vi "TransferCavityLock_InfIntegral_SlowCavityLock.vi"() -> ()   [LabVIEW 2016]
uses:
  <vilib>/DAQmx/read.llb/DAQmx Read (Analog 1D Wfm NChan NSamp Duration).vi
  <vilib>/Analysis/baseanly.llb/Mean (DBL).vi
  <vilib>/DAQmx/create/channels.llb/DAQmx Create Channel (AI-Voltage-Basic).vi
  <vilib>/DAQmx/configure/timing.llb/DAQmx Timing (Sample Clock).vi
  <vilib>/DAQmx/configure/trigger.llb/DAQmx Start Trigger (Digital Edge).vi
  <vilib>/DAQmx/miscellaneous.llb/DAQmx Fill In Error Info.vi
  <vilib>/Waveform/WDTOps.llb/WDT Get Waveform Subset DBL.vi
  <vilib>/measure/mamon.llb/Waveform Peak Detection for 1 Chan.vi
  <vilib>/addons/control/pid/pid.llb/PID (DBL).vi
  <vilib>/measure/NI_MAPro.lvlib
  <vilib>/Analysis/NI_AALBase.lvlib
  <vilib>/addons/control/pid/NI_PID_pid.lvlib
  <vilib>/gmath/NI_Gmath.lvlib
panel:
  in  "Limit for cavity lock":bool
  in  "Polarity 2":i8=1 min=-1 max=1 step=2
  in  "Polarity 1":i8=1 min=-1 max=1 step=2
  out "Integral for cavity lock":dbl=0.008257081575736186 format="%0.5f V"
  out "Cavity scan offset Output":dbl=3.2082570815757308 min=0.0 step=0.01 format="%.5f V"
  in  "Cavity scan offset":dbl=3.1999999999999944 min=0.0 step=0.01 format="%.5f V"
  in  "OK Button 2":bool
  out "Error Signal for cavity lock":dbl(graph)=1.2838768115943822
  in  "Setpoint for cavity lock":dbl=1950.0 min=0.0 step=0.1 format="%.2f"
  in  "I Factor for cavity lock":dbl=5e-05 min=0.0 step=1e-05 format="%.5f"
  out "Peak Loc2":dbl(graph)=2256.4418259303447
  out "Peak Loc1":dbl(graph)=1948.7161231884056
  out "PZT Output":dbl(graph)=4.680700597703368
  out "Noise Std":dbl=0.03727411119636263 format="%0.3f V"
  out "size(s)":i32=100
  out "Histogram":dynamicdata(graph)=[{"t0"=timestamp(-0.09499999999999997 s since 1904-01-01), "dt"=0.01, "Y"=[0.6724792202903564, 0.8210147212924623, 2.0418544555563467, 2.399967444273753, 2.6421006582360897, 3.8191936353555187, 6.9191091939405664, 9.895923412654003, 9.585626646861932, 10.44733602596319, 14.545288067308965, 9.500167865463462, 6.621020825491134, 7.961909800290967, 3.825297834026838, 3.17316594264088, 2.0886533120364623, 1.9238399479108381, 0.4415370372254382, 0.6745139531807962], "attributes"=variant("NI_ChannelName"=variant(string " (Histogram)"), "NI_ExpIsRelativeTime"=variant(bool TRUE), "NI_ExpStartTimeStamp"=variant(timestamp timestamp(0 s since 1904-01-01)), "NI_ExpTimeStamp"=variant(timestamp timestamp(0 s since 1904-01-01)), "NI_ExpXDimension"=variant(string "BIN"), "NI_OriginalChannelName"=variant(string ""))}]
  out "Integral":dbl=-0.31929940229663345 format="%0.3f V"
  in  "I Factor":dbl=0.06 min=0.0 step=1e-05 format="%.3f"
  in  "Proportional":T1={"Proportional gain (Kc)"=0.005, "Integral time (Ti, min)"=0.1, "Derivative time (Td, min)"=0.0} {"Derivative time (Td, min)" min=0.0 step=0.1 format="%.2f"; "Integral time (Ti, min)" min=0.0 step=0.1 format="%.2f"; "Proportional gain (Kc)" min=0.0 step=0.1 format="%.3f"}
  out "P Array":dbl[](array[numeric])=[0.06979206777050706, -0.06757152621814555, 0.0253521126760603, 0.04560439560439988, -0.038277511961723576, 0.036986301369879016, -0.04494569757727618, 0.02419763085957527, 0.018115942028984477, -0.011801242236018084, -0.012648809523824411, -0.04897959183674061, 0.023401360544227146, -0.007827788649706235, -0.02202273314389913, 0.011767925561031234, 0.011688311688303088, -0.023990241257791922, -0.02863234846175544, 0.06390977443608392, -0.052721088435390584, 0.057637600494757635, 0.03265306122450795, 0.08333333333334281, -0.014731645166421004, -9.5174645480256e-05, 0.00201465201466533, -0.1062769282757472, 0.06927854753941176, -0.010158730158735807, 0.03962304562004704, -0.08253968253968935, -0.058129809300780266, -0.06380952380952465, 0.056462585033997925, 0.010964912280698513, 0.006632653061231508, 0.09833024118738365, -0.03107769423559148, 0.02233831742027803, -0.031212484993986322, 0.005787389582692981, 0.03754094230284011, 0.08456760630672022, 0.01198879551820653, -0.020408163265315693, 0.002782931354346374, 0.005864661654143788, -0.029870129870133155, 0.009480715363082481, -0.07006573673240268, -0.01208244491826349, -0.018367346938788387, -0.04200542005420971, -0.041410488245915644, 0.0015444015443932813, 0.009890109890108079, -0.05175983436853926, -0.017460317460304964, -0.015971606033730268, 0.0018796992481213692, -0.03761904761904589, -0.03679653679652972, 0.040224785566394416, 0.022408963585434094, 0.009680795395070163, 0.11904761904760619, 0.01256157635468469, 0.00023060071485758726, -0.027777777777785673, -0.03336594911937141, 0.034962406015054626, -0.040259740259742216, -0.030677655677649796, 0.01959183673470477, -0.02309092651145761, -0.0007963051441350899, -0.0, -0.0, -0.0, 0.0, -0.0, -0.0, 0.0, 0.0, 0.0, -0.0, 0.0, -0.0, 0.0, 0.0, 0.0, 0.0, -0.0, 0.0, -0.0, -0.0, -0.0, 0.0, -0.0]
  out "Full?":bool=TRUE
  in  "PZT Value":dbl=5.000000000000002 min=0.0 step=0.01 format="%.2f V"
  out "Error Signal":dbl(graph)=-0.003649068322971516
  in  "Output Range":cluster{"Output high":dbl, "Output low":dbl}={"Output high"=1.0, "Output low"=-1.0} {"Output low" min=0.0 format="%.2f"; "Output high" min=0.0 max=1.0 format="%.2f"}
  out "P Output":dbl=-1.824534161485758e-05 format="%0.3f V"
  in  "Setpoint":dbl=115.0 min=0.0 step=0.1 format="%.2f"
  out "dt out (s)":dbl=0.4020000190939754 format="%.3f"
  out "Number of Peaks":i32=8
  out "Average Spacing":dbl(graph)=115.00364906832297
  out "Current Value":dbl=115.00364906832297 format="%0.2f"
  out "Spcaing":dbl[](array[numeric])=[58.58871915393655, 185.2243243243243, 71.53859649122808, 165.22807017543857, 82.54838709677426, 146.8474462365591, 95.04999999999995]
  out "Locations":dbl[](array[numeric])=[128.58695652173913, 187.17567567567568, 372.4, 443.93859649122805, 609.1666666666666, 691.7150537634409, 838.5625, 933.6125]
  out "error out 2":errorcluster
  in  "Peak Thres":dbl=-0.15 format="%.2f"
  in  "width 2":i32=3 min=3
  out "Waveform Graph 2":waveform(dbl)(graph)={"t0"=timestamp(3654386435.809387 s since 1904-01-01), "dt"=9.999999999999999e-05, "Y"=array[1000 elements], "attributes"=variant("NI_ChannelName"=variant(string "Voltage_1"), "NI_UnitDescription"=variant(string "Volts"))}
  out "Rate":dbl=5.0 format="%#_g Hz"
  in  "OK Button":bool
  in  "Physical channels":tag="Dev1/ao0"
  out "Waveform Graph":waveform(dbl)[](graph)=[{"t0"=timestamp(3654386435.7613373 s since 1904-01-01), "dt"=9.999999999999999e-05, "Y"=array[1500 elements], "attributes"=variant("NI_ChannelName"=variant(string "Voltage_0"), "NI_UnitDescription"=variant(string "Volts"))}, {"t0"=timestamp(3654386435.7613873 s since 1904-01-01), "dt"=9.999999999999999e-05, "Y"=array[1500 elements], "attributes"=variant("NI_ChannelName"=variant(string "Voltage_1"), "NI_UnitDescription"=variant(string "Volts"))}]
  in  "error in":errorcluster
  in  "stop":bool
  # "锁定：\n1. Proportional gain (Kc)设置为0.005\n2. Integral time (Ti, min)设置为0.10\n3. Derivative time (Td, min)设置为0.00\n4. I Factor设置为0.06\n5. 调节PZT电压使得Current Value在Setpoint附近（Error Signal0.1以内）\n6. 点击Lock Off，状态变为Lock On \n\n解锁：\n1. 点击Lock On\n2. 点击Stop"
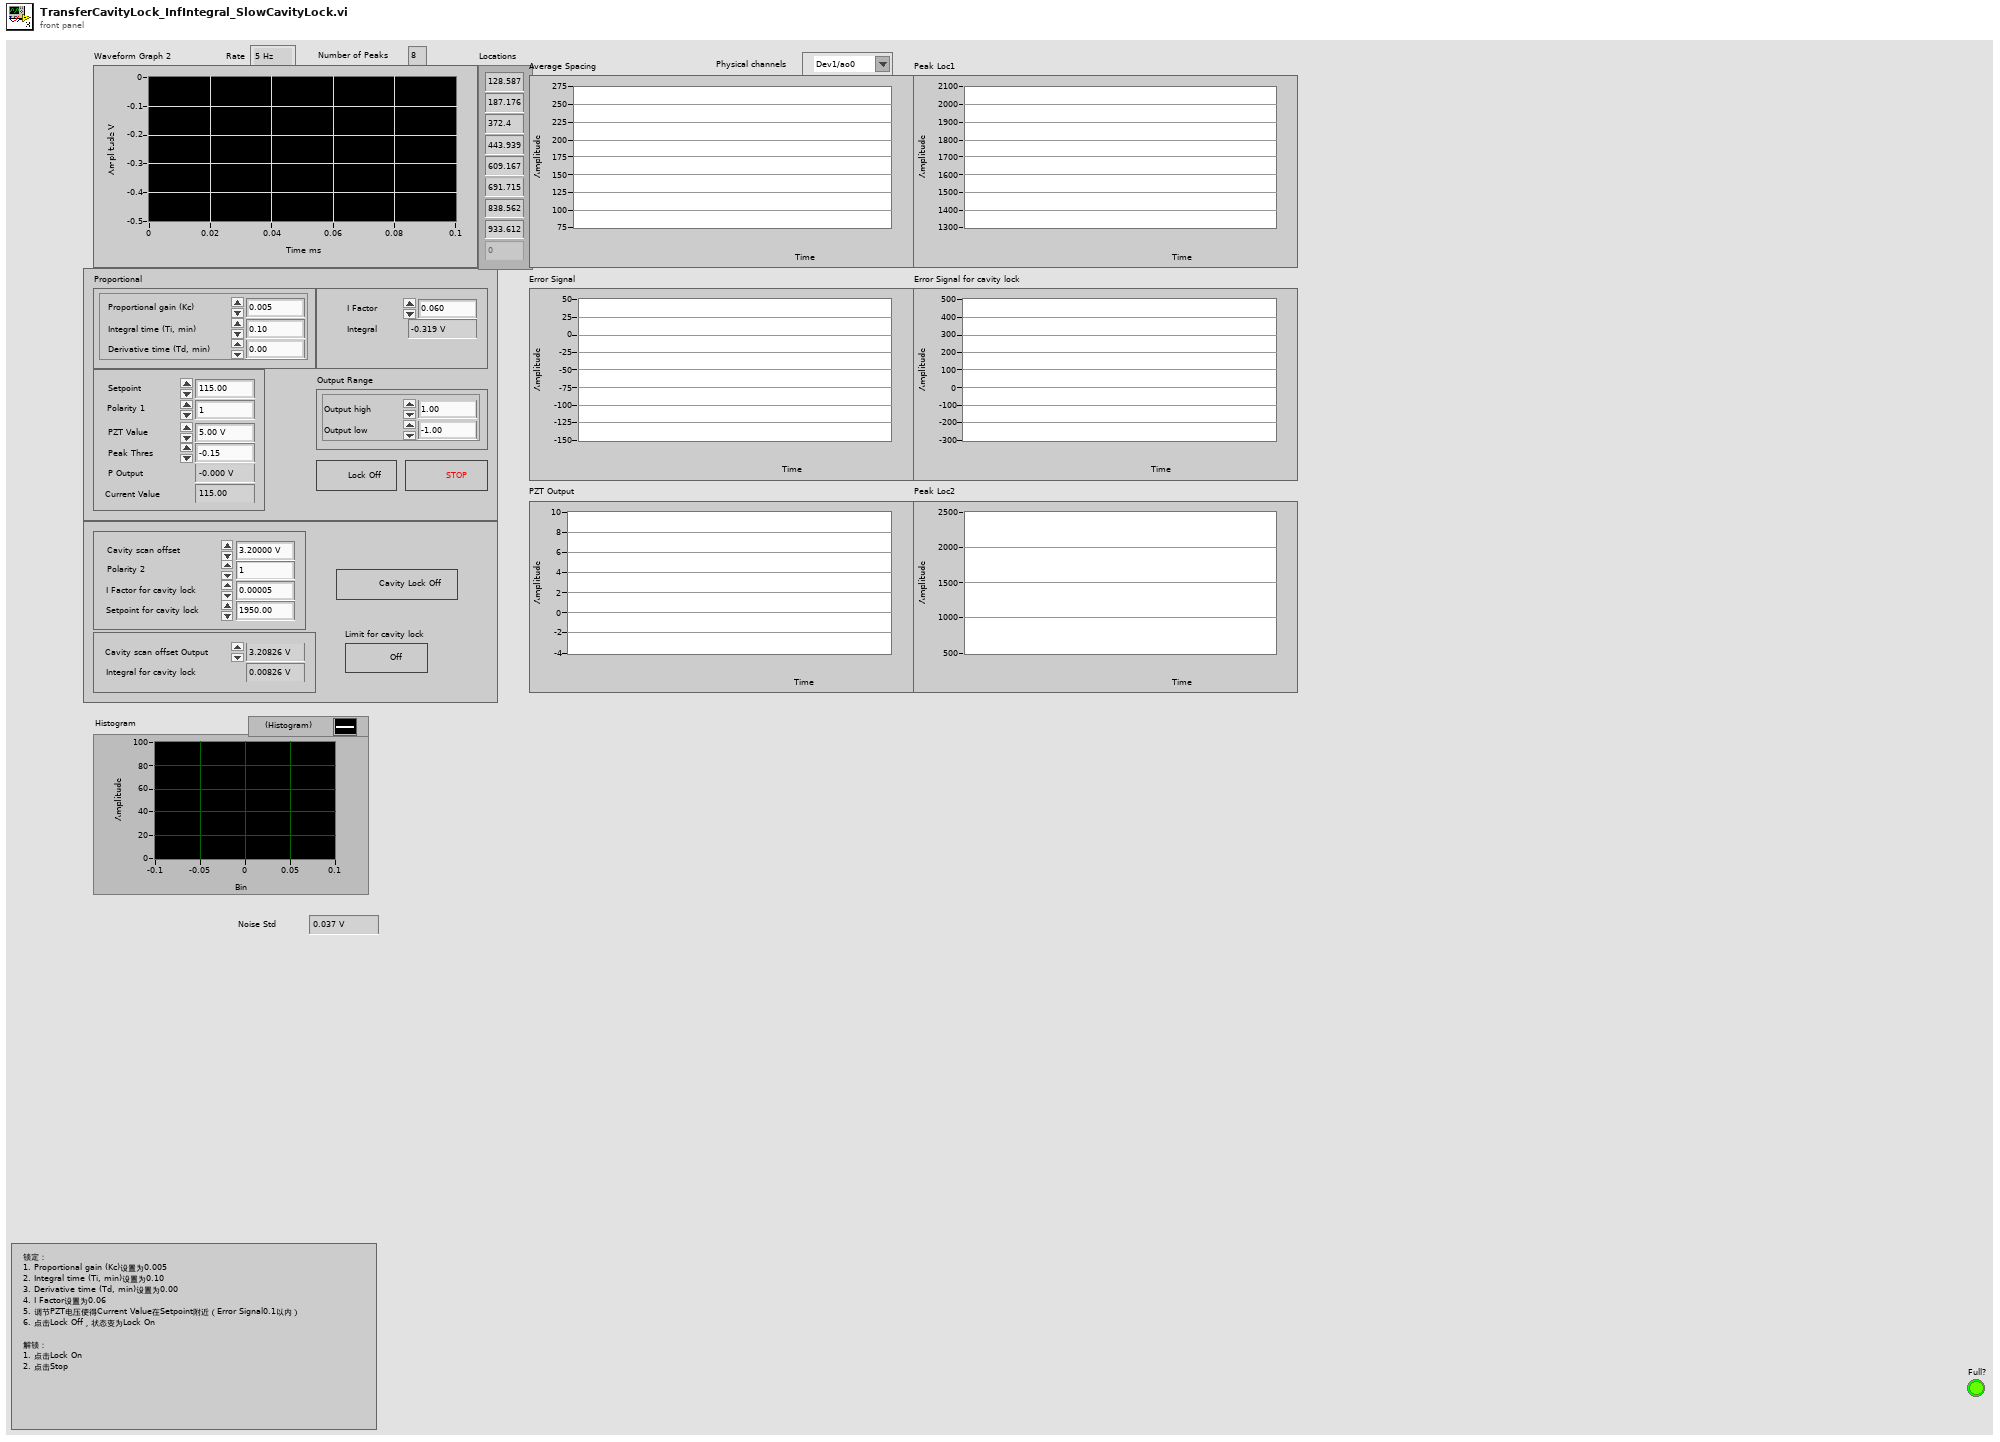
[diagram p1: front panel]
types:
  T1 = cluster{"Proportional gain (Kc)":dbl, "Integral time (Ti, min)":dbl, "Derivative time (Td, min)":dbl}
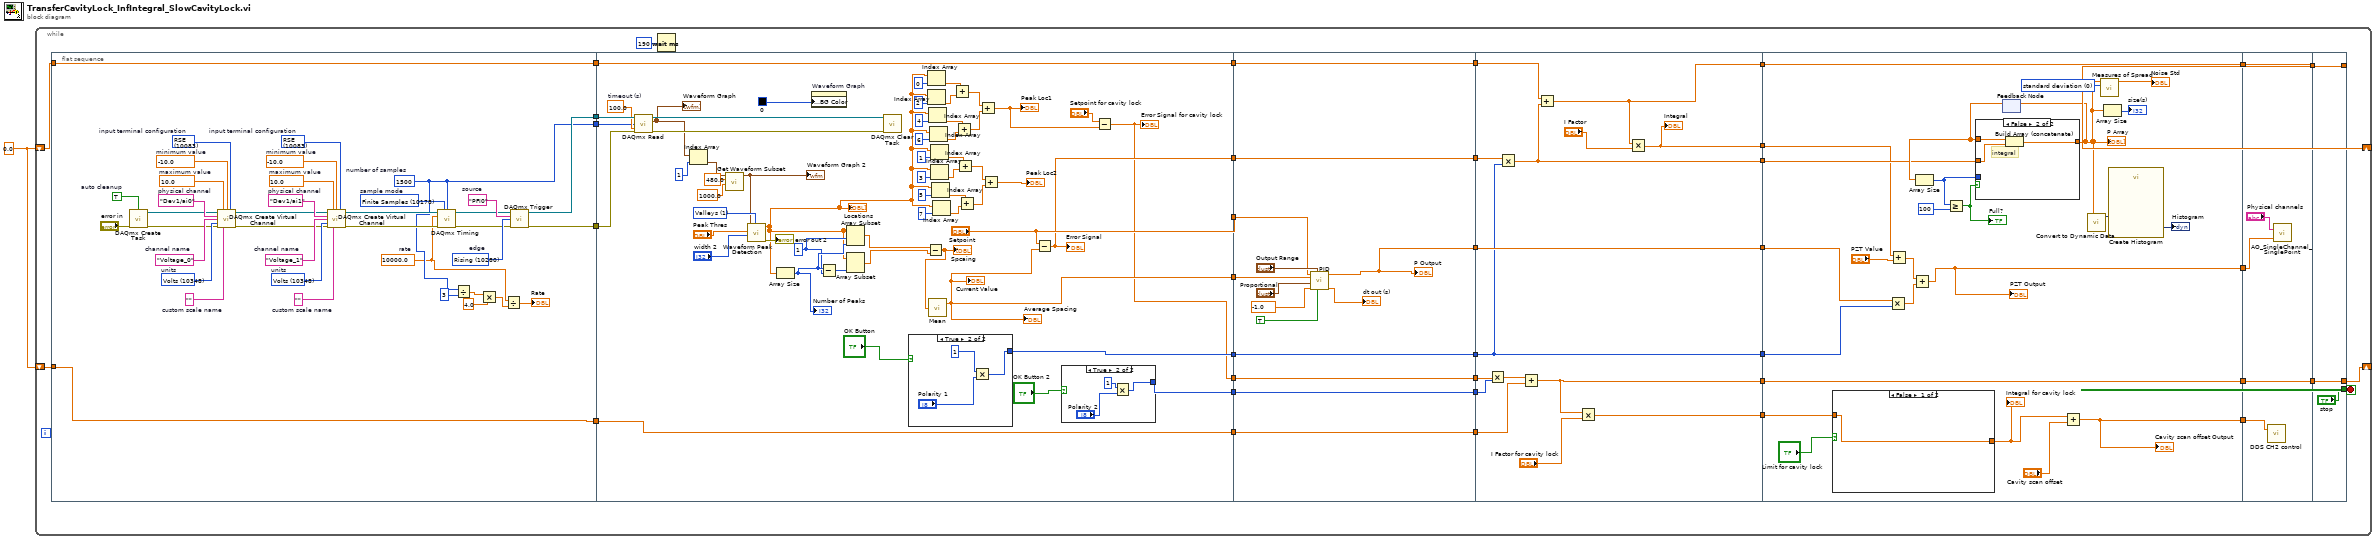
[diagram p0: block diagram]
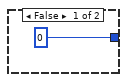
[diagram p2: hidden frame]
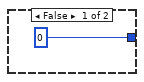
[diagram p3: hidden frame]
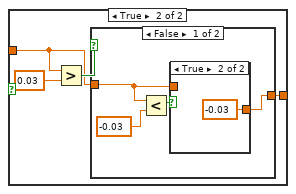
[diagram p4: hidden frame]
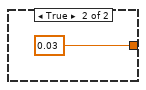
[diagram p6: hidden frame]
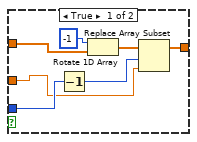
[diagram p7: hidden frame]
diagram:
  w1 = 0.0
  n1 = while {
    shift-right: [w17] -> _
    shift-left: w1 -> [w23]
    shift-right: [w2] -> _
    shift-left: w1 -> [w14]
    stop <- w36 stop-if-true
    n2 = flat-sequence {
      tunnel: [w51] -> w40
      tunnel: [w50] -> w39
      tunnel: [w49] -> w38
      tunnel: [w42] -> w24
      tunnel: w23 -> [w42]
      tunnel: [w41] -> w15
      tunnel: w14 -> [w41]
      tunnel: w40 -> [w132]
      tunnel: w39 -> [w131]
      tunnel: w38 -> [w129]
      tunnel: [w109] -> w35
      tunnel: [w111] -> w34
      tunnel: ["Setpoint"] -> w32
      tunnel: [w108] -> w31
      tunnel: w24 -> [w107]
      tunnel: [w107] -> w21
      tunnel: w15 -> [w80]
      tunnel: [w82] -> w12
      tunnel: [w81] -> w10
      tunnel: [w80] -> w9
      tunnel: w35 -> [w154]
      tunnel: [w147] -> w30
      tunnel: [w157] -> w28
      tunnel: w34 -> [w157]
      tunnel: w32 -> [w155]
      tunnel: [w150] -> w27
      tunnel: w31 -> [w150]
      tunnel: [w148] -> w22
      tunnel: w21 -> [w148]
      tunnel: [w146] -> w13
      tunnel: w12 -> [w146]
      tunnel: [w145] -> w11
      tunnel: w10 -> [w145]
      tunnel: w9 -> [w144]
      tunnel: [w144] -> w8
      tunnel: w30 -> [w172]
      tunnel: [w172] -> w29
      tunnel: w28 -> [w170]
      tunnel: w27 -> [w171]
      tunnel: [w169] -> w26
      tunnel: [w170] -> w25
      tunnel: w22 -> [w168]
      tunnel: [w167] -> w20
      tunnel: [w166] -> w16
      tunnel: w13 -> [w164]
      tunnel: w11 -> [w163]
      tunnel: w8 -> [w162]
      tunnel: [w159] -> w7
      tunnel: [w158] -> w3
      tunnel: w29 -> [w196]
      tunnel: [w179] -> w33
      tunnel: w26 -> [w190]
      tunnel: w25 -> [w191]
      tunnel: w20 -> [w189]
      tunnel: [w189] -> w18
      tunnel: w16 -> [w188]
      tunnel: w7 -> [w175]
      tunnel: [w177] -> w6
      tunnel: [w176] -> w4
      tunnel: w3 -> [w176]
      tunnel: w33 -> [w223]
      tunnel: [w222] -> w19
      tunnel: w18 -> [w222]
      tunnel: w6 -> [w221]
      tunnel: [w220] -> w5
      tunnel: w4 -> [w220]
      tunnel: ["stop"] -> w36
      tunnel: w19 -> [w226]
      tunnel: [w226] -> w17
      tunnel: w5 -> [w225]
      tunnel: [w225] -> w2
      frame #0 {
        w78 = 10280 items=["Rising"=10280, "Falling"=10171]  # edge
        w77 = "PFI0"  # source
        w75 = 10178 items=["Finite Samples"=10178, "Continuous Samples"=10123, "Hardware Timed Single Point"=12522]  # sample mode
        w49 = 1500  # number of samples
        w45 = 10000.0  # rate
        w72 = 10083 items=["default"=-1, "RSE"=10083, "NRSE"=10078, "Differential"=10106, "Pseudodifferential"=12529]  # input terminal configuration
        w71 = 10348 items=["Volts"=10348, "From Custom Scale"=10065]  # units
        w70 = "Voltage_1"  # channel name
        w68 = ""  # custom scale name
        w67 = -10.0  # minimum value
        w66 = 10.0  # maximum value
        w65 = "Dev1/ai1"  # physical channel
        w63 = 10083 items=["default"=-1, "RSE"=10083, "NRSE"=10078, "Differential"=10106, "Pseudodifferential"=12529]  # input terminal configuration
        w62 = 10348 items=["Volts"=10348, "From Custom Scale"=10065]  # units
        w61 = "Voltage_0"  # channel name
        w59 = ""  # custom scale name
        w58 = -10.0  # minimum value
        w57 = 10.0  # maximum value
        w56 = "Dev1/ai0"  # physical channel
        w54 = TRUE  # auto cleanup
        n3 = call <vilib>:"DAQmx Create Task.vi"("auto cleanup"=w54, "error in"="error in") -> ("task out"=w55:refnum<k21>, "error out"=w53:errorcluster)  [unwired: 12 in]
        n4 = call-poly <vilib>:"DAQmx Create Virtual Channel.vi"("task in"=w55, "maximum value"=w57, "minimum value"=w58, "input terminal configuration"=w63, "physical channels"=w56, "name to assign"=w61, "units"=w62, "error in"=w53, "custom scale name"=w59) -> ("task out"=w64:refnum<k21>, "error out"=w60:errorcluster)  [unwired: 5 in]
        n5 = call-poly <vilib>:"DAQmx Create Virtual Channel.vi"("task in"=w64, "maximum value"=w66, "minimum value"=w67, "input terminal configuration"=w72, "physical channels"=w65, "name to assign"=w70, "units"=w71, "error in"=w60, "custom scale name"=w68) -> ("task out"=w74:refnum<k21>, "error out"=w69:errorcluster)  [unwired: 5 in]
        n6 = call-poly <vilib>:"DAQmx Timing.vi"("task/channels in"=w74, "sample mode"=w75, "samples per channel"=w49, "rate"=w45, "error in"=w69) -> ("task out"=w76:refnum<k21>, "error out"=w73:errorcluster)  [unwired: 9 in]
        n7 = Divide(x=w49, y=3) -> (x/y=w47:dbl)
        n8 = Multiply(x=w47, y=4.0) -> (x*y=w44:dbl)
        n9 = Divide(x=w45, y=w44) -> (x/y=→"Rate":dbl)
        n10 = call-poly <vilib>:"DAQmx Trigger.vi"("task/channels in"=w76, "source"=w77, "edge"=w78, "error in"=w73) -> ("task out"=w51:refnum<k21>, "error out"=w50:errorcluster)  [unwired: 10 in]
      }
      frame #1 {
        w116 = 1 ("index")
        w123 = u16 1 items=["Peaks", "Valleys"] ("peaks/valleys")
        w130 = 100.0  # timeout (s)
        n11 = call-poly <vilib>:"DAQmx Read.vi"("task/channels in"=w132, "duration"=w129, "timeout"=w130, "error in"=w131) -> ("task out"=w134:refnum<k21>, "data"=w128:waveform(dbl)[], "error out"=w133:errorcluster)  [unwired: 9 in]
        "Waveform Graph" <- w128
        n12 = Index Array(array=w128, index=1) -> (element=w126:waveform(dbl))
        n13 = call-poly <vilib>:"Get Waveform Subset.vi"("duration"=1000.0, "start samples/time"=480.0, "waveform in"=w126) -> ("waveform out"=w119:waveform(dbl))  [unwired: 3 in, 3 out]
        "Waveform Graph 2" <- w119
        n14 = call-poly <vilib>:"Waveform Peak Detection.vi"("peaks/valleys"=w123, "width"="width 2", "threshold"="Peak Thres", "Signal In"=w119) -> ("error out"=→"error out 2":errorcluster, "Locations"=w86:dbl[])  [unwired: 3 in, 3 out]
        "Locations" <- w86
        n15 = Array Size(array=w86) -> (size(s)=w118:i32)
        "Number of Peaks" <- w118
        n16 = property on="Waveform Graph" class="WFGraph (strict)"("Plot Area:Colors:BG Color"=u32 0) -> ()  [unwired: 2 in, 2 out]
        n17 = Subtract(x=w118, y=w116) -> (x-y=w117:i32)
        n18 = Array Subset(array=w86, index=w116, length=w118) -> (w113:dbl[])
        n19 = Array Subset(array=w86, length=w117) -> (w112:dbl[])  [unwired: 1 in]
        n20 = call <vilib>:"DAQmx Clear Task.vi"("task in"=w134, "error in"=w133) -> ()  [unwired: 13 in, 1 out]
        n21 = case shown="True" "OK Button" {
          tunnel: [0 w141] -> w111
          frame False {
          }
          frame True {
            n22 = Multiply(x=1, y="Polarity 1") -> (x*y=w141:i32)
          }
        }
        n23 = Subtract(x=w113, y=w112) -> (x-y=w115:dbl[])
        "Spcaing" <- w115
        n24 = Index Array(array=w86, index=0) -> (element=w102:dbl)
        n25 = Index Array(array=w86, index=2) -> (element=w101:dbl)
        n26 = Index Array(array=w86, index=4) -> (element=w100:dbl)
        n27 = call-poly <vilib>:"Mean.vi"("X"=w115) -> ("mean"=w109:dbl)  [unwired: 1 out]
        "Current Value" <- w109
        "Average Spacing" <- w109
        n28 = Index Array(array=w86, index=6) -> (element=w99:dbl)
        n29 = Index Array(array=w86, index=1) -> (element=w92:dbl)
        n30 = Index Array(array=w86, index=3) -> (element=w91:dbl)
        n31 = Index Array(array=w86, index=5) -> (element=w90:dbl)
        n32 = Index Array(array=w86, index=7) -> (element=w89:dbl)
        n33 = Add(x=w102, y=w101) -> (x+y=w98:dbl)
        n34 = Add(x=w100, y=w99) -> (x+y=w97:dbl)
        n35 = Add(x=w92, y=w91) -> (x+y=w88:dbl)
        n36 = Add(x=w90, y=w89) -> (x+y=w87:dbl)
        n37 = Add(x=w98, y=w97) -> (x+y=w79:dbl)
        "Peak Loc1" <- w79
        n38 = Add(x=w88, y=w87) -> (x+y=→"Peak Loc2":dbl)
        n39 = Subtract(x="Setpoint", y=w109) -> (x-y=w108:dbl)
        "Error Signal" <- w108
        n40 = case shown="True" "OK Button 2" {
          tunnel: [0 w138] -> w81
          frame False {
          }
          frame True {
            n41 = Multiply(x=1, y="Polarity 2") -> (x*y=w138:i32)
          }
        }
        n42 = Subtract(x="Setpoint for cavity lock", y=w79) -> (x-y=w82:dbl)
        "Error Signal for cavity lock" <- w82
      }
      frame #2 {
        n43 = call-poly <vilib>:"PID.vi"("reinitialize? (F)"=TRUE, "output range"="Output Range", "dt (s)"=-1.0, "PID gains"="Proportional", "process variable"=w154, "setpoint"=w155) -> ("dt out (s)"=→"dt out (s)":dbl, "output"=w147:dbl)  [unwired: 4 in]
        "P Output" <- w147
      }
      frame #3 {
        n44 = Multiply(x=w164, y=w163) -> (x*y=w161:dbl)
        n45 = Multiply(x=w171, y=w170) -> (x*y=w169:dbl)
        n46 = Add(x=w161, y=w162) -> (x+y=w158:dbl)
        n47 = Add(x=w168, y=w169) -> (x+y=w167:dbl)
        n48 = Multiply(x=w158, y="I Factor for cavity lock") -> (x*y=w159:dbl)
        n49 = Multiply(x=w167, y="I Factor") -> (x*y=w166:dbl)
        "Integral" <- w166
      }
      frame #4 {
        w182 = 0 items=["standard deviation", "range", "mean absolute deviation", "interquartile range"] ("type")
        # "integral"
        n50 = case shown="False" "Limit for cavity lock" {
          tunnel: w175 -> [w198 w200]
          tunnel: [w198 w199] -> w174
          frame False {
          }
          frame True {
            n51 = Greater?(x=w200, y=0.03) -> (0:w201:bool)
            n52 = case shown="False" w201 {
              tunnel: [w204 0.03 ("y")] -> w199
              tunnel: w200 -> [w203 _]
              frame False {
                n53 = Less?(x=w203, y=-0.03) -> (x < y?=w205:bool)
                n54 = case shown="True" w205 {
                  tunnel: [w207 -0.03 ("y")] -> w204
                  tunnel: w203 -> [w207 _]
                  frame False {
                  }
                  frame True {
                  }
                }
              }
              frame True {
              }
            }
          }
        }
        "Integral for cavity lock" <- w174
        n55 = Multiply(x=w196, y=w191) -> (x*y=w197:dbl)
        n56 = Add(x=w188, y="PZT Value") -> (x+y=w186:dbl)
        n57 = Add(x=w186, y=w197) -> (x+y=w179:dbl)
        "PZT Output" <- w179
        n58 = feedback #1() -> (w195:dbl[])  [unwired: 1 in]
        n59 = Array Size(array=w195) -> (size(s)=w194:i32)
        n60 = Greater Or Equal?(x=w194, y=100 ("I Size 1")) -> (x >= y?=w193:bool)
        "Full?" <- w193
        n61 = case shown="False" w193 {
          tunnel: [w210 w219] -> w183
          tunnel: w195 -> [w214 w218]
          tunnel: w194 -> [w212 _]
          tunnel: w190 -> [w211 w217]
          frame True {
            n62 = Decrement(x=w212) -> (x-1=w213:i32)
            n63 = Rotate 1D Array(1:w214, 2:-1 ("n")) -> (0:w216:dbl[])
            n64 = Replace Array Subset(array=w216, new element=w211, index=w213) -> (w210:dbl[])
          }
          frame False {
            n65 = Build Array (concatenate)(w218, w217) -> (w219:dbl[])
          }
        }
        "P Array" <- w183
        n66 = feedback-in #1(w183) -> ()
        n67 = Add(x=w174, y="Cavity scan offset") -> (x+y=w177:dbl)
        "Cavity scan offset Output" <- w177
        n68 = call "Convert to Dynamic Data"("Array"=w183) -> ("Dynamic Data Type"=w185:dynamicdata)  [unwired: 3 in]
        n69 = call <vilib>:"Measures of Spread.vi"("type"=w182, "x array"=w183) -> ("spread value"=→"Noise Std":dbl)  [unwired: 8 in, 1 out]
        n70 = Array Size(array=w183) -> (size(s)=→"size(s)":i32)
        n71 = call "Create Histogram"("Signal"=w185) -> ("Histogram"=→"Histogram":dynamicdata)  [unwired: 9 in, 1 out]
      }
      frame #5 {
        n72 = call "DDS CH2 control.vi"("DC Offset (0.00 V)"=w221) -> ()  [unwired: 2 in]
        n73 = call "AO_SingleChannel_SinglePoint.vi"("voltage"=w223, "physical channels"="Physical channels") -> ()  [unwired: 2 in]
      }
      frame #6 {
      }
    }
    n74 = Wait (ms)(milliseconds to wait=u32 190) -> ()  [unwired: 1 out]
  }
